vi "mainPLC.vi"(8 "Error In":errorcluster, 11 "plcUDE":T1) -> (0 "Error Out":errorcluster)   [LabVIEW 2018]
uses:
  controls/plcUDE.ctl
  controls/plcData.ctl
  controls/modbusDriverSelectorEnum.ctl
  controls/openModbusConnectionCluster.ctl
  controls/readRegisterModbusCluster.ctl
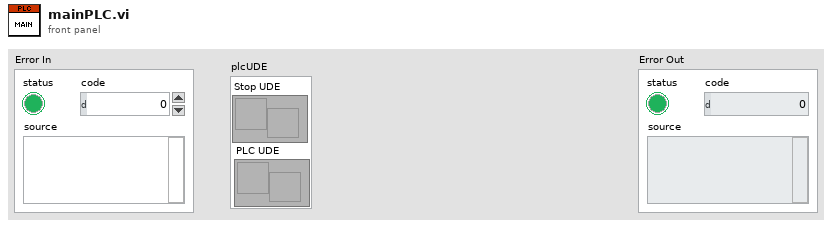
[diagram p1: front panel]
types:
  T1 = typedef "plcUDE.ctl" = cluster{"Stop UDE":refnum<user-event>, "PLC UDE":refnum<user-event>}
  T2 = enum32{"Invalid", "Standard", "Closed", "Hidden", "Minimized", "Maximized"}
  T3 = enum32{"invalid app kind", "Development System", "Run Time System", "Student Edition", "Embedded LabVIEW", "Evaluation", "Custom"}
  T4 = typedef "openModbusConnectionCluster.ctl" = cluster{"IP Address":string, "Timeout (ms)":i32, "Port (502)":u16}
  T5 = typedef "modbusDriverSelectorEnum.ctl" = enum16{"open", "write single holding registers", "read holding registers", "close"}
  T6 = typedef "plcData.ctl" = cluster{"IP Address":string, "Timeout":i32, "Port [502]":u16, "isSimulation?":bool, "Model Number":u16}
  T7 = cluster{"Core":cluster{"Current VI Reference":refnum<vi>, "Close Panel on Exit?":bool}, "plcUDE":T1, "PLC Data":T6, "Address":u16, "Registry":i32, "Setting-Registry":u16, "DB file path":path}
  T8 = cluster{"Current VI Reference":refnum<vi>, "Close Panel on Exit?":bool}
  T9 = typedef "pathCluster.ctl" = cluster{"src Folder Path":path, "Controller Module Path":path, "UI Module Path":path, "Model Select Module Path":path, "Barcode Printer Module Path":path, "Barcode Scanner Module Path":path, "Database Module Path":path, "Report Generation Path":path, "Simulation Path":path, "subVIs Folder Path":path, "info Folder Path":path, "config file Path":path, "cutomerLogo Path":path}
  T10 = typedef "readRegisterModbusCluster.ctl" = cluster{"Starting Address":u16, "Number of Inputs":u16}
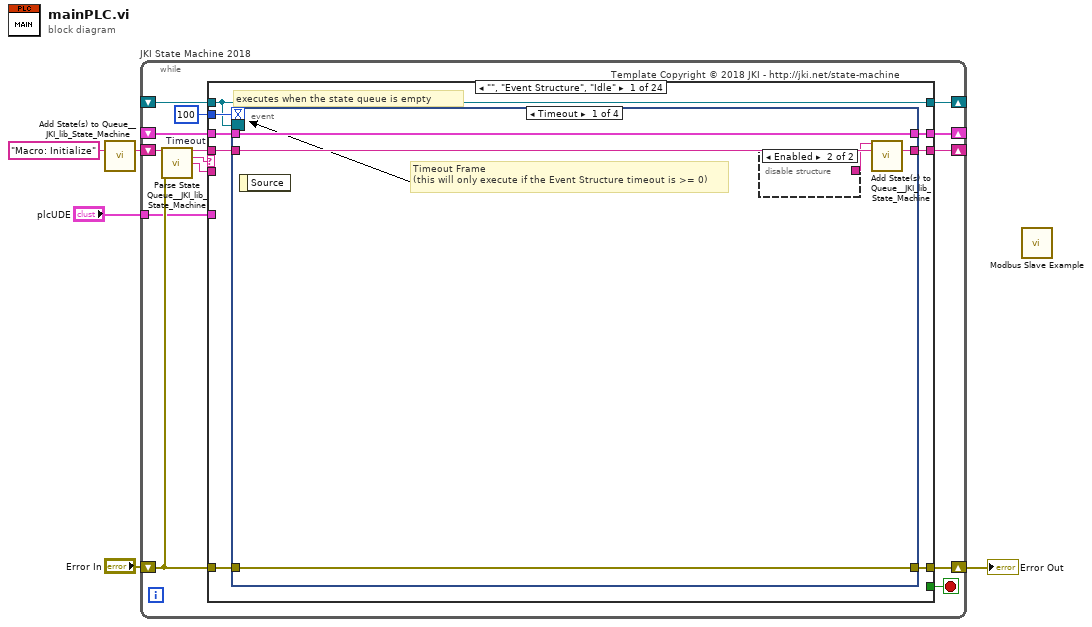
[diagram p0: block diagram]
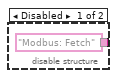
[diagram p2: hidden frame]
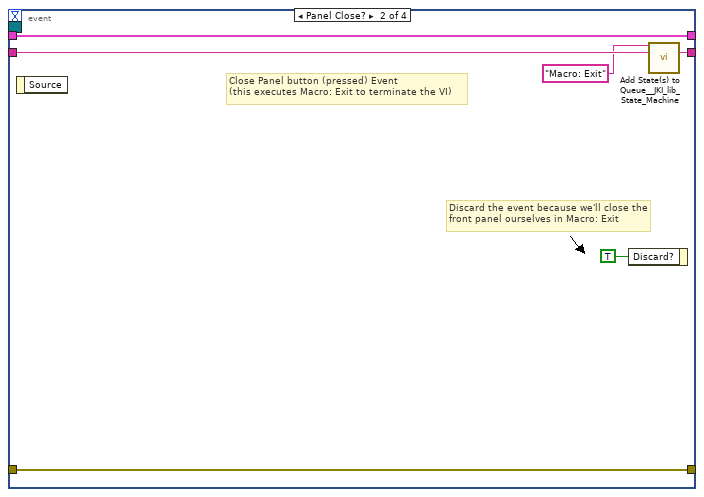
[diagram p3: hidden frame]
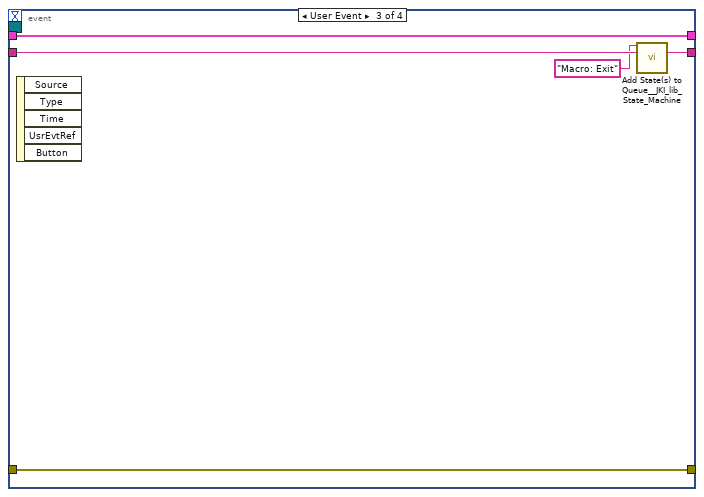
[diagram p4: hidden frame]
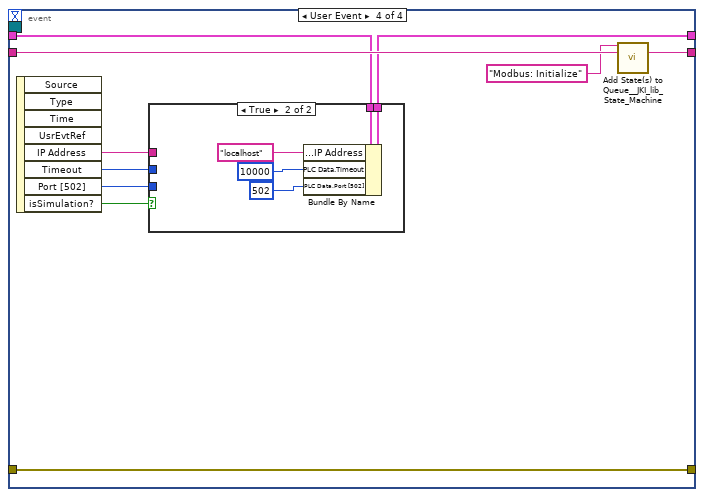
[diagram p5: hidden frame]
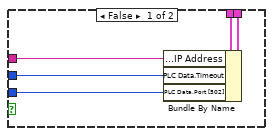
[diagram p6: hidden frame]
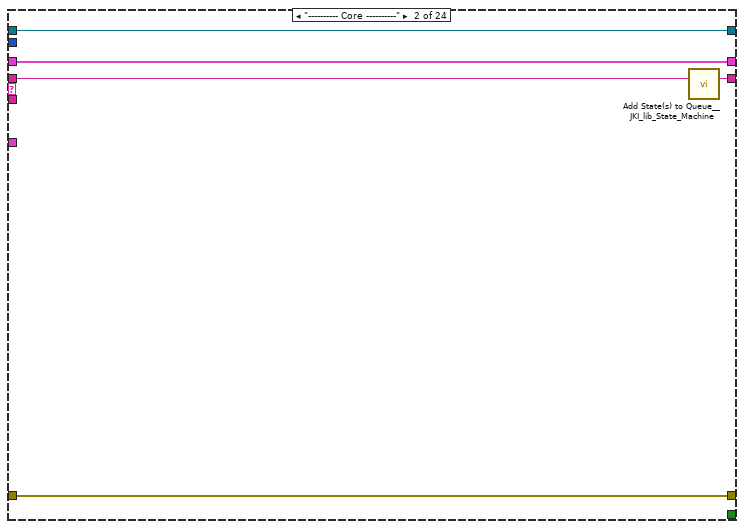
[diagram p7: hidden frame]
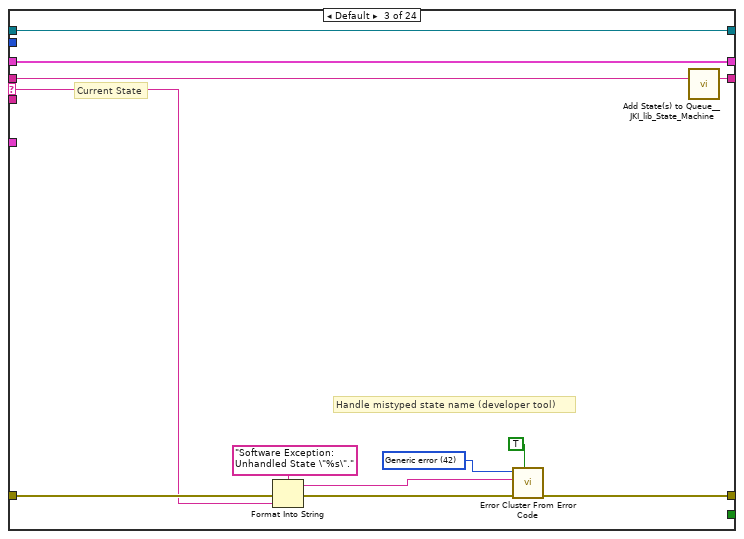
[diagram p8: hidden frame]
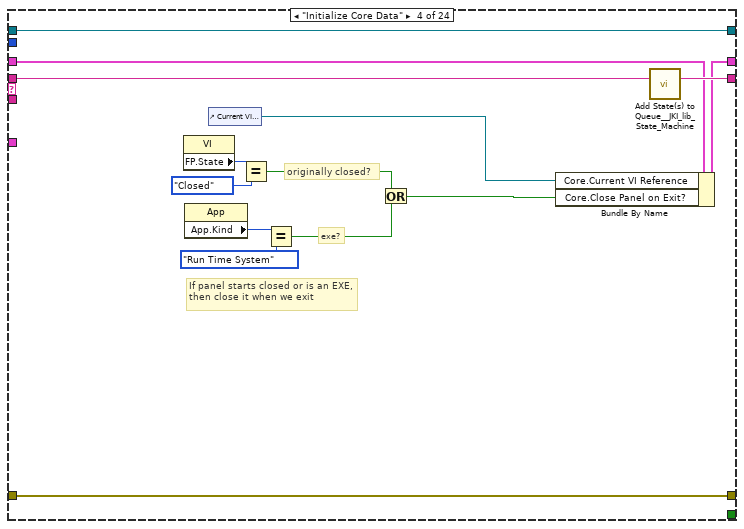
[diagram p9: hidden frame]
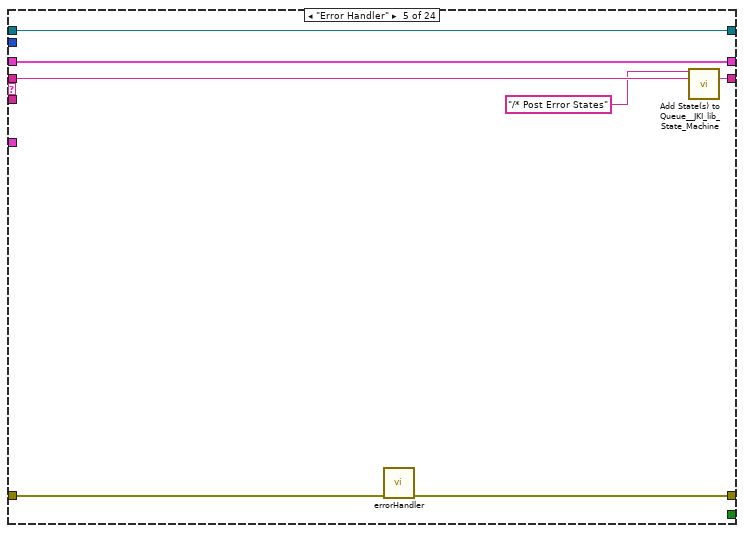
[diagram p10: hidden frame]
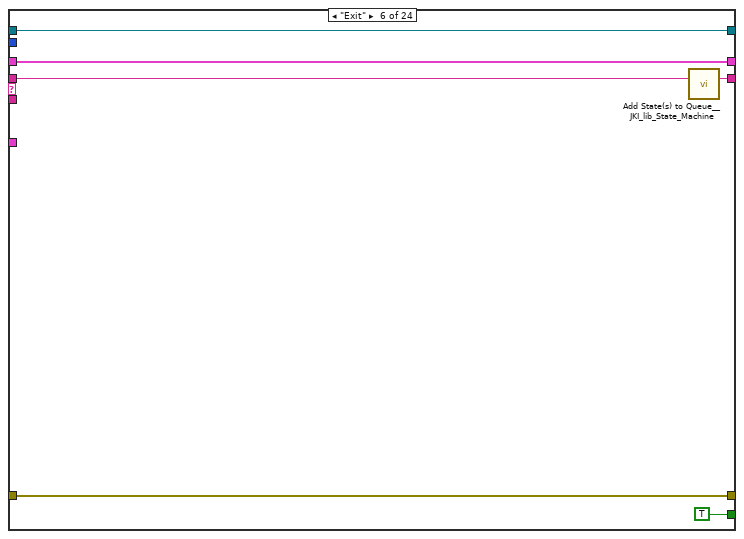
[diagram p11: hidden frame]
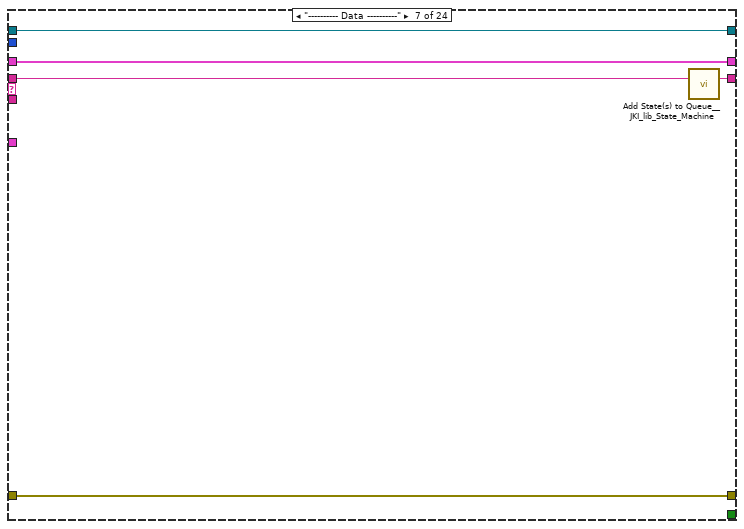
[diagram p12: hidden frame]
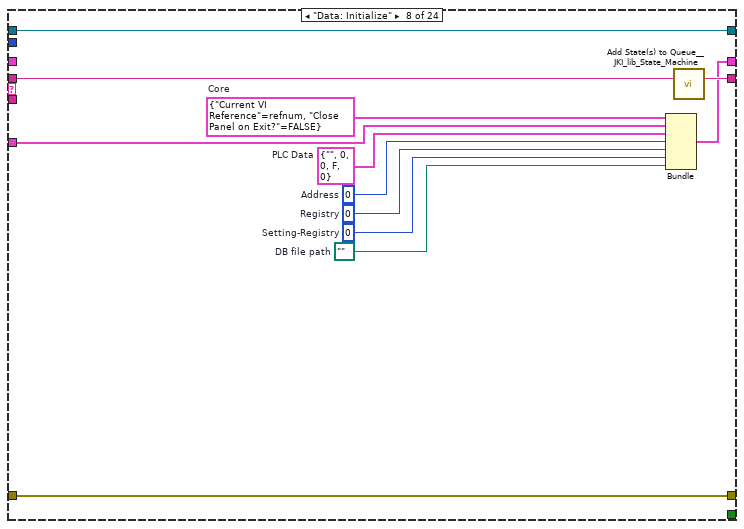
[diagram p13: hidden frame]
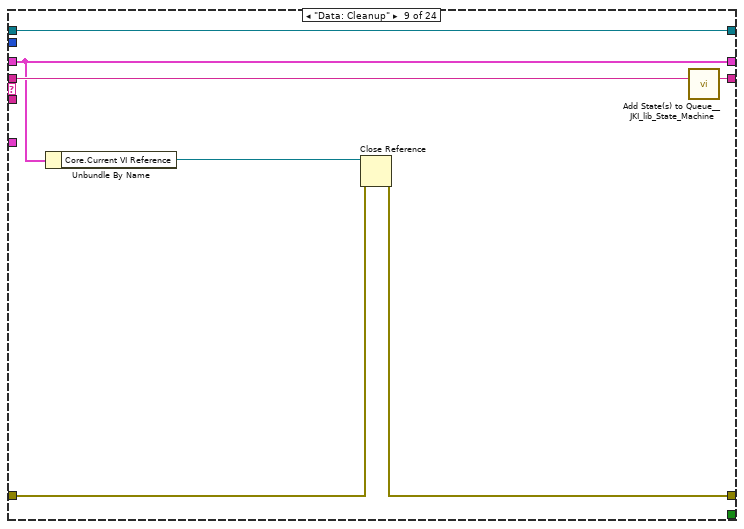
[diagram p14: hidden frame]
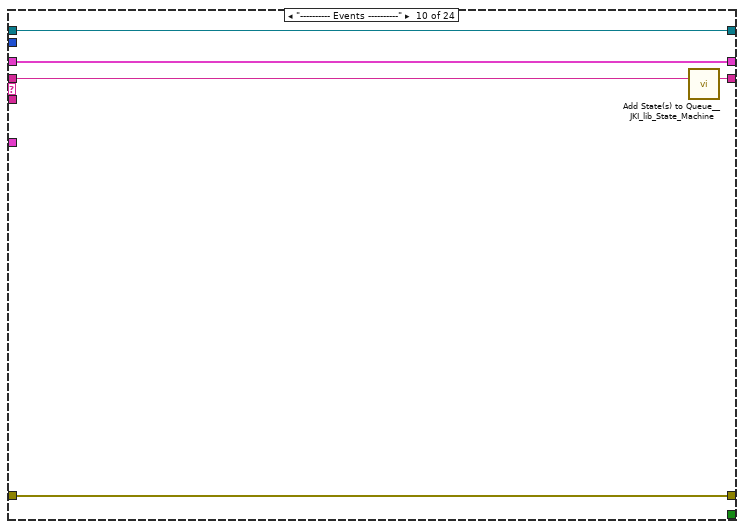
[diagram p15: hidden frame]
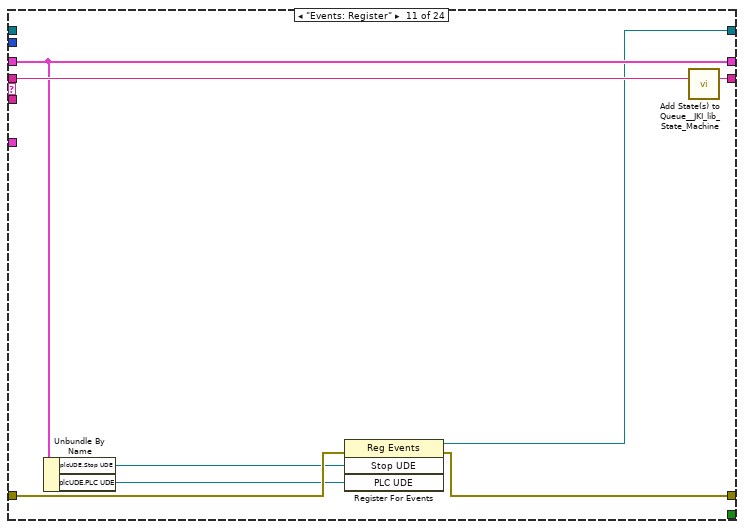
[diagram p16: hidden frame]
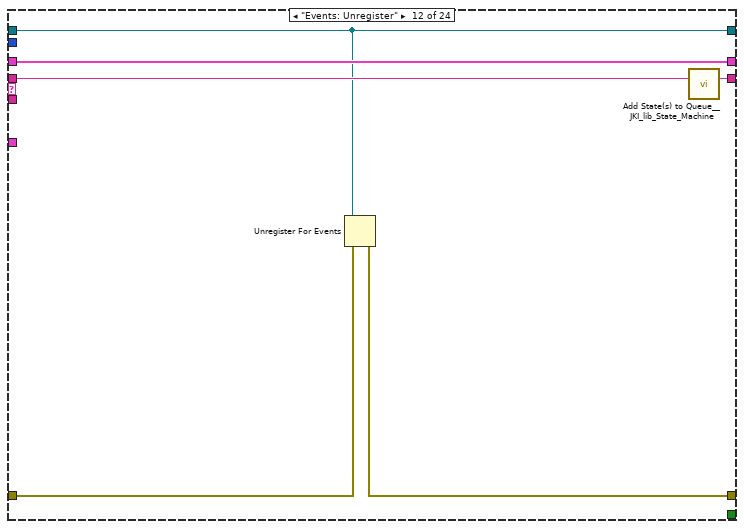
[diagram p17: hidden frame]
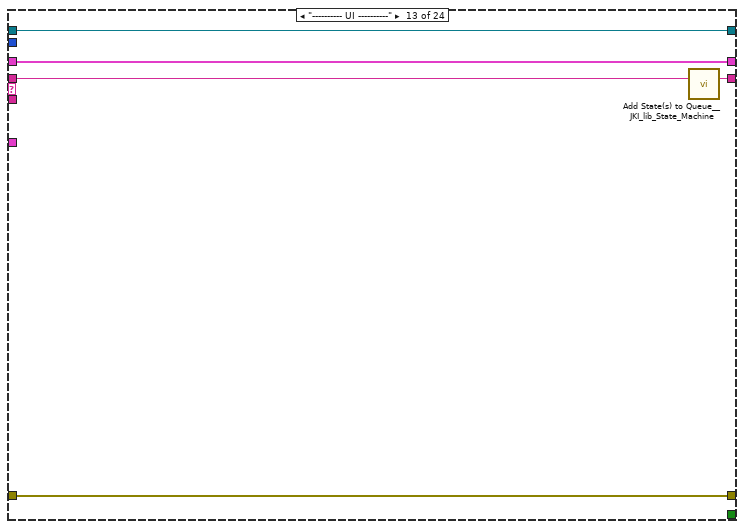
[diagram p18: hidden frame]
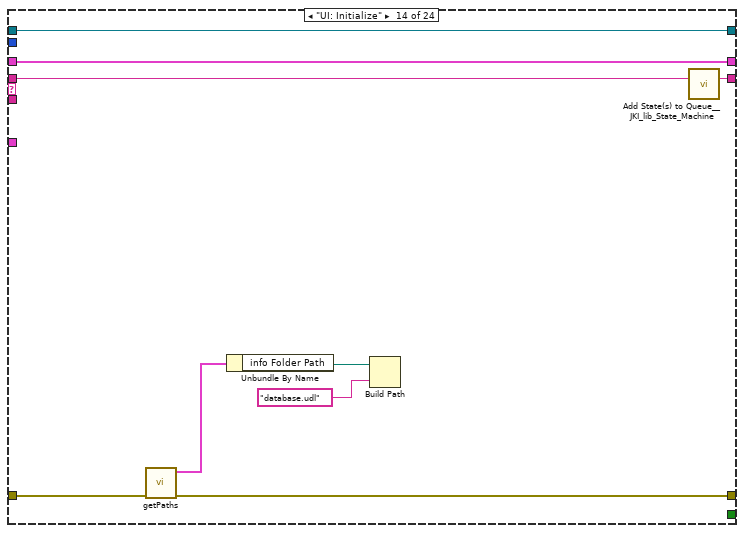
[diagram p19: hidden frame]
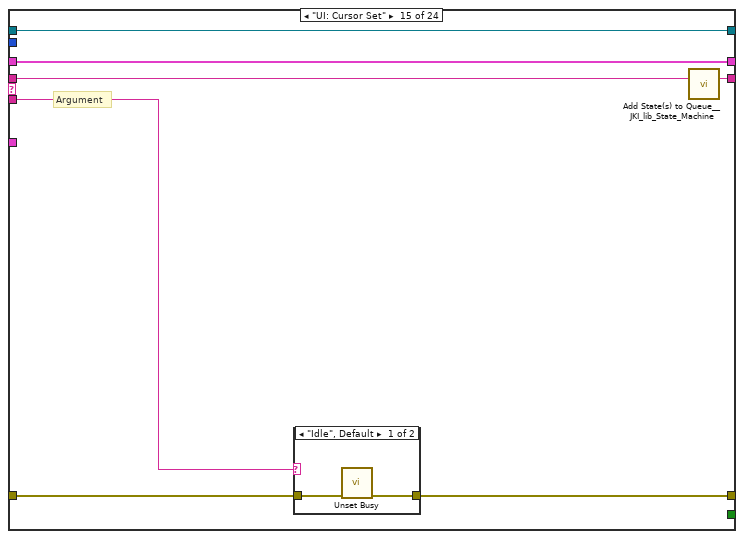
[diagram p20: hidden frame]
diagram:
  n1 = call <vilib>:"Add State(s) to Queue__JKI_lib_State_Machine.vi"("State(s) in (\"\")"="Macro: Initialize") -> ("States Out"=w5:string)  [unwired: 14 in]
  n2 = while "JKI State Machine 2018" {
    shift-right: [w12] -> _
    shift-left: _ -> [w11]
    shift-right: [w15] -> w2
    shift-left: "Error In" -> [w9]
    shift-right: [w14] -> _
    shift-left: w5 -> [w16]
    shift-right: [w8] -> _
    shift-left: _ -> [w7]
    tunnel: "plcUDE" -> [w6]
    stop <- w13 stop-if-true
    w10 = 100  # Timeout
    # "Template Copyright © 2018 JKI - http://jki.net/state-machine"
    n3 = call <vilib>:"Parse State Queue__JKI_lib_State_Machine.vi"("State Queue"=w16, "Error In (no error)"=w9) -> ("Remaining States"=w18:string, "Current State"=w19:string, "Arguments"=w17:string)  [unwired: 11 in]
    n4 = case shown="\"\", \"Event Structure\", \"Idle\"" w19 {
      selector: w19 -> [_ _ w71 _ _ _ _ _ _ _ _ _ _ _ _ _ _ _ _ _ _ _ _ _]
      tunnel: w18 -> [w27 w69 w75 w95 w102 w108 w113 w125 w132 w137 w145 w151 w156 w165 w172 w184 w254 w260 w271 w276 w288 w306 w315 w334]
      tunnel: w17 -> [_ _ _ _ _ _ _ _ _ _ _ _ _ _ w167 w178 _ _ _ _ _ _ _ _]
      tunnel: w11 -> [w25 w66 w73 w88 w100 w106 w110 _ w127 w134 w141 w149 w153 w162 w170 w180 w251 w257 w268 w273 w282 w296 w312 w332]
      tunnel: [w24 w67 w77 w92 w96 w105 w111 w122 w128 w135 w143 w146 w154 w160 w168 w181 w252 w258 w269 w274 w284 w302 w310 w327] -> w15
      tunnel: w9 -> [w23 w67 w76 w92 w97 w105 w111 w122 w129 w135 w142 w147 w154 w161 w169 w182 w252 w258 w269 w274 w285 w303 w311 w330]
      tunnel: [w26 w68 w74 w94 w101 w107 w112 w124 w131 w136 w144 w150 w155 w164 w171 w183 w253 w259 w270 w275 w287 w305 w314 w333] -> w14
      tunnel: [_ _ _ _ _ TRUE _ _ _ _ _ _ _ _ _ _ _ _ _ _ _ _ _ _] -> w13
      tunnel: [w22 w66 w73 w93 w100 w106 w110 w123 w127 w134 w141 w149 w153 w162 w170 w180 w251 w257 w268 w273 w282 w295 w312 w332] -> w12
      tunnel: w10 -> [w21 _ _ _ _ _ _ _ _ _ _ _ _ _ _ _ _ _ _ _ _ _ _ _]
      tunnel: [w20 w65 w70 w82 w98 w103 w109 w120 w126 w133 w138 w148 w152 w163 w166 w177 w250 w255 w261 w272 w286 w304 w313 w331] -> w8
      tunnel: w7 -> [w20 w65 w70 w82 w98 w103 w109 w120 w126 w133 _ w148 w152 w163 w166 w177 w250 w255 w261 w272 w286 w304 w313 w331]
      tunnel: w6 -> [_ _ _ _ _ _ _ w119 _ _ _ _ _ _ _ _ _ _ _ _ _ _ _ _]
      frame "", "Event Structure", "Idle" {
        # "executes when the state queue is empty"
        n5 = event shown="[0] Timeout" {
          selector: w20 -> [_ _ _ _]
          dyn-events: _ -> [_ _ _ _]
          timeout: w21 -> [_ _ _ _]
          tunnel: w27 -> [w32 w39 w42 w53]
          tunnel: [w31 w38 w41 w52] -> w26
          tunnel: w25 -> [w29 w36 w44 w45]
          tunnel: [w30 w37 w43 w54] -> w24
          tunnel: w23 -> [w30 w37 w43 w54]
          tunnel: [w29 w36 w44 w46] -> w22
          event Timeout {
            # "Timeout Frame\n(this will only execute if the Event Structure timeout is >= 0)"
            n6 = event-data() -> ()  [unwired: 1 in, 1 out]
            n7 = disable-structure shown="Enabled" {
              disable-tunnel: ["Modbus: Fetch" ("State(s) in Front (\"\")") _] -> w28
              frame Disabled {
              }
              frame Enabled {
              }
            }
            n8 = call <vilib>:"Add State(s) to Queue__JKI_lib_State_Machine.vi"("State(s) in Front (\"\")"=w28, "State(s) in (\"\")"=w32) -> ("States Out"=w31:string)  [unwired: 13 in]
          }
          event Panel Close? {
            # "Discard the event because we'll close the front panel ourselves in Macro: Exit"
            # "Close Panel button (pressed) Event\n(this executes Macro: Exit to terminate the VI)"
            n9 = event-data() -> ()  [unwired: 1 in, 1 out]
            n10 = event-data("Discard?"=TRUE) -> ()  [unwired: 1 in, 1 out]
            n11 = call <vilib>:"Add State(s) to Queue__JKI_lib_State_Machine.vi"("State(s) in Front (\"\")"="Macro: Exit", "State(s) in (\"\")"=w39) -> ("States Out"=w38:string)  [unwired: 13 in]
          }
          event User Event {
            n12 = event-data() -> ()  [unwired: 1 in, 5 out]
            n13 = call <vilib>:"Add State(s) to Queue__JKI_lib_State_Machine.vi"("State(s) in Front (\"\")"="Macro: Exit" ("State(s) in Front (\"\")"), "State(s) in (\"\")"=w42) -> ("States Out"=w41:string)  [unwired: 13 in]
          }
          event User Event {
            n14 = event-data() -> ("IP Address"=w47:string, "Timeout"=w48:i32, "Port [502]"=w49:u16, "isSimulation?"=w50:bool)  [unwired: 1 in, 4 out]
            n15 = case shown="True" w50 {
              tunnel: w49 -> [w57 _]
              tunnel: w48 -> [w58 _]
              tunnel: w47 -> [w59 _]
              tunnel: w45 -> [w56 w64]
              tunnel: [w55 w63] -> w46
              frame False {
                n16 = Bundle By Name(cluster=w56, "PLC Data.IP Address"=w59, "PLC Data.Timeout"=w58, "PLC Data.Port [502]"=w57) -> (w55:T7)
              }
              frame True {
                n17 = Bundle By Name(cluster=w64, "PLC Data.IP Address"="localhost", "PLC Data.Timeout"=10000, "PLC Data.Port [502]"=u16 502) -> (w63:T7)
              }
            }
            n18 = call <vilib>:"Add State(s) to Queue__JKI_lib_State_Machine.vi"("State(s) in Front (\"\")"="Modbus: Initialize" ("State(s) in (\"\")"), "State(s) in (\"\")"=w53) -> ("States Out"=w52:string)  [unwired: 13 in]
          }
        }
      }
      frame "---------- Core ----------" {
        n19 = call <vilib>:"Add State(s) to Queue__JKI_lib_State_Machine.vi"("State(s) in (\"\")"=w69) -> ("States Out"=w68:string)  [unwired: 14 in]
      }
      frame Default {
        w80 = 42 items=["No error", "Argument error", "Memory is full", "Out of zone", "End of file", "File already open", "Generic file I/O error", "File not found", "File permission error", "Disk is full", "Duplicate path", "Too many files open", "System feature not enabled", "Resource file not found", "Cannot add resource", "Resource not found", "Image not found", "Image memory error", "Pen does not exist", "Config type invalid", "Config token not found", "Config parse error", "Config memory error", "Bad external code format", "Bad external code offset", "External code not present", "Null window", "Destroy window error", "Null menu", "Print aborted", "Bad print record", "Print driver error", "Windows error during printing", "Memory error during printing", "Print dialog error", "Generic print error", "Invalid device refnum", "Device not found", "Device parameter error", "Device unit error", "Cannot open device", "Device call aborted", "Generic error", "Cancelled by user", "Object ID too low", "Object ID too high", "Object not in heap", "Unknown heap", "Unknown object (invalid DefProc)", "Unknown object (DefProc not in table)", "Message out of range", "Invalid (null) method", "Unknown message", "Manager call not supported", "Bad address", "Network operation in progress", "Network operation timed out", "Connection is busy", "Network attribute not supported", "Network error", "Address in use", "System out of memory", "Connection aborted", "Connection refused", "Not connected", "Already connected", "Connection closed", "Initialization error (interapplication manager)", "Bad occurrence", "Wait on unbound occurrence handler", "Occurrence queue overflow", "Datalog type conflict", "Unused", "Unrecognized type (interapplication manager)", "Memory corrupt", "Failed to make temporary DLL", "Old CIN version", "Drag socket not found", "Failed to load drop-object", "Failed to register OLE object", "Failed to release OLE object", "Format specifier type mismatch", "Unknown format specifier", "Too few format specifiers", "Too many format specifiers", "Scan failed", "Newer CIN version", "Error converting to variant", "Runtime menu error", "Password tampered", "Variant attribute not found", "Incompatible variant data type", "Event data is not available", "Event Store is not present", "Occurrence is not found", "Event Queue is not created", "Event info is not available", "Refnum passed is NULL", "Error retrieving Class GUID", "Error retrieving CoClass GUID", "Error retrieving TypeLib GUID.", "Bad built application magic bytes.", "Specific driver is different from the specific driver associated with the Logical Name.", "There is no session opened to the class driver.", "Max Error", "MAX - Error with config objects", "MAX - Error loading configuration", "MAX - Group not supported"]
        # "Current State"
        # "Handle mistyped state name (developer tool)"
        n20 = Format Into String(format string="Software Exception: Unhandled State \"%s\"." ("message"), error in=w76, w71) -> (resulting string=w79:string, error out=w78:errorcluster)  [unwired: 1 in]
        n21 = call <vilib>:"Error Cluster From Error Code.vi"("show call chain? (False)"=TRUE, "error in (no error)"=w78, "error message (\"\")"=w79, "error code (0)"=w80) -> ("error out"=w77:errorcluster)  [unwired: 5 in]
        n22 = call <vilib>:"Add State(s) to Queue__JKI_lib_State_Machine.vi"("State(s) in (\"\")"=w75) -> ("States Out"=w74:string)  [unwired: 14 in]
      }
      frame "Initialize Core Data" {
        # "originally closed?"
        # "exe?"
        # "If panel starts closed or is an EXE, then close it when we exit"
        n23 = property class="VI"() -> ("FP.State"=w85:T2)  [unwired: 2 in, 2 out]
        n24 = property class="App"() -> ("App.Kind"=w91:T3)  [unwired: 2 in, 2 out]
        n25 = control-ref of="Current VI Reference"() -> (w86:refnum<vi>)
        n26 = Equal?(x=w85, y=T2."Closed" ("Front Panel Window:State")) -> (x = y?=w83:bool)
        n27 = Equal?(x=w91, y=T3."Run Time System" ("Application:Kind")) -> (x = y?=w89:bool)
        n28 = Or(x=w83, y=w89) -> (x .or. y?=w87:bool)
        n29 = Bundle By Name(cluster=w88, "Core.Current VI Reference"=w86, "Core.Close Panel on Exit?"=w87) -> (w93:T7)
        n30 = call <vilib>:"Add State(s) to Queue__JKI_lib_State_Machine.vi"("State(s) in (\"\")"=w95) -> ("States Out"=w94:string)  [unwired: 14 in]
      }
      frame "Error Handler" {
        n31 = call "errorHandler.vi"("Error In"=w97) -> ("Error Out"=w96:errorcluster)  [unwired: 10 in]
        n32 = call <vilib>:"Add State(s) to Queue__JKI_lib_State_Machine.vi"("State(s) in Front (\"\")"="/* Post Error States", "State(s) in (\"\")"=w102) -> ("States Out"=w101:string)  [unwired: 13 in]
      }
      frame "Exit" {
        n33 = call <vilib>:"Add State(s) to Queue__JKI_lib_State_Machine.vi"("State(s) in (\"\")"=w108) -> ("States Out"=w107:string)  [unwired: 14 in]
      }
      frame "---------- Data ----------" {
        n34 = call <vilib>:"Add State(s) to Queue__JKI_lib_State_Machine.vi"("State(s) in (\"\")"=w113) -> ("States Out"=w112:string)  [unwired: 14 in]
      }
      frame "Data: Initialize" {
        w114 = path ""  # DB file path
        w115 = u16 0  # Setting-Registry
        w116 = 0  # Registry
        w117 = u16 0  # Address
        w118 = T6 {"IP Address"="", "Timeout"=0, "Port [502]"=0, "isSimulation?"=FALSE, "Model Number"=0}  # PLC Data
        w121 = T8 {"Current VI Reference"=refnum, "Close Panel on Exit?"=FALSE}  # Core
        n35 = Bundle("Core"=w121, "plcUDE"=w119, "PLC Data"=w118, "Address"=w117, "Registry"=w116, "Setting-Registry"=w115, "DB file path"=w114) -> (w123:T7)  [unwired: 1 in]
        n36 = call <vilib>:"Add State(s) to Queue__JKI_lib_State_Machine.vi"("State(s) in (\"\")"=w125) -> ("States Out"=w124:string)  [unwired: 14 in]
      }
      frame "Data: Cleanup" {
        n37 = Unbundle By Name(w127) -> ("Core.Current VI Reference"=w130:refnum<vi>)
        n38 = Close Reference(reference=w130, error in (no error)=w129) -> (error out=w128:errorcluster)
        n39 = call <vilib>:"Add State(s) to Queue__JKI_lib_State_Machine.vi"("State(s) in (\"\")"=w132) -> ("States Out"=w131:string)  [unwired: 14 in]
      }
      frame "---------- Events ----------" {
        n40 = call <vilib>:"Add State(s) to Queue__JKI_lib_State_Machine.vi"("State(s) in (\"\")"=w137) -> ("States Out"=w136:string)  [unwired: 14 in]
      }
      frame "Events: Register" {
        n41 = Unbundle By Name(w141) -> ("plcUDE.Stop UDE"=w140:refnum<user-event>, "plcUDE.PLC UDE"=w139:refnum<user-event>)
        n42 = register-events(error in=w142, w140, w139) -> (reference out=w138:refnum<event-registration>, error out=w143:errorcluster)  [unwired: 1 in]
        n43 = call <vilib>:"Add State(s) to Queue__JKI_lib_State_Machine.vi"("State(s) in (\"\")"=w145) -> ("States Out"=w144:string)  [unwired: 14 in]
      }
      frame "Events: Unregister" {
        n44 = Unregister For Events(event registration refnum=w148, error in=w147) -> (error out=w146:errorcluster)
        n45 = call <vilib>:"Add State(s) to Queue__JKI_lib_State_Machine.vi"("State(s) in (\"\")"=w151) -> ("States Out"=w150:string)  [unwired: 14 in]
      }
      frame "---------- UI ----------" {
        n46 = call <vilib>:"Add State(s) to Queue__JKI_lib_State_Machine.vi"("State(s) in (\"\")"=w156) -> ("States Out"=w155:string)  [unwired: 14 in]
      }
      frame "UI: Initialize" {
        n47 = call "getPaths.vi"("Error In"=w161) -> ("Error Out"=w160:errorcluster, "Application Path Cluster"=w159:T9)  [unwired: 9 in]
        n48 = Unbundle By Name(w159) -> ("info Folder Path"=w158:path)
        n49 = Build Path(base path=w158, name or relative path="database.udl") -> ()  [unwired: 1 out]
        n50 = call <vilib>:"Add State(s) to Queue__JKI_lib_State_Machine.vi"("State(s) in (\"\")"=w165) -> ("States Out"=w164:string)  [unwired: 14 in]
      }
      frame "UI: Cursor Set" {
        # "Argument"
        n51 = case shown="\"Idle\", Default" w167 {
          tunnel: w169 -> [w174 w176]
          tunnel: [w173 w175] -> w168
          frame "Idle", Default {
            n52 = call <vilib>:"Unset Busy.vi"("error in (no error)"=w174) -> ("error out"=w173:errorcluster)  [unwired: 10 in]
          }
          frame "Busy" {
            n53 = call <vilib>:"Set Busy.vi"("error in (no error)"=w176) -> ("error out"=w175:errorcluster)  [unwired: 9 in, 1 out]
          }
        }
        n54 = call <vilib>:"Add State(s) to Queue__JKI_lib_State_Machine.vi"("State(s) in (\"\")"=w172) -> ("States Out"=w171:string)  [unwired: 14 in]
      }
      frame "UI: Front Panel State" {
        # "Argument"
        n55 = Unbundle By Name(w180) -> ("Core.Current VI Reference"=w179:refnum<vi>)
        n56 = case shown="\"Open\", \"Standard\", Default" w178 {
          tunnel: w182 -> [w190 w205 w216 w229 w242]
          tunnel: [w192 w206 w218 w231 w244] -> w181
          tunnel: w179 -> [w191 w203 w217 w230 w243]
          frame "Open", "Standard", Default {
            w185 = T2."Hidden" ("State")
            n57 = property class="VI"(reference=w191, error in=w190) -> (reference out=w188:refnum<vi>, error out=w189:errorcluster, "FP.State"=w187:T2)
            n58 = Not Equal?(x=w187, y=w185) -> (x != y?=w186:bool)
            n59 = case shown="True" w186 {
              tunnel: [w196 w198] -> w192
              tunnel: w189 -> [w195 w198]
              tunnel: w188 -> [w194 _]
              tunnel: w185 -> [w193 _]
              frame True {
                n60 = invoke class="VI" method="FP.Open"(reference=w194, error in=w195, "Activate"=TRUE, "State"=w193) -> (error out=w196:errorcluster)  [unwired: 1 in, 4 out]
              }
              frame False {
              }
            }
          }
          frame "Close", "Closed" {
            n61 = property class="VI"(reference=w203, error in=w205) -> (reference out=w202:refnum<vi>, error out=w204:errorcluster, "FP.State"=w200:T2)
            n62 = Not Equal?(x=w200, y=T2."Closed" ("Front Panel Window:State")) -> (x != y?=w199:bool)
            n63 = case shown="True" w199 {
              tunnel: [w207 w210] -> w206
              tunnel: w204 -> [w207 w209]
              tunnel: w202 -> [_ w208]
              frame False {
              }
              frame True {
                n64 = invoke class="VI" method="FP.Close"(reference=w208, error in=w209) -> (error out=w210:errorcluster)  [unwired: 1 in, 2 out]
              }
            }
          }
          frame "Hidden", "Hide" {
            w211 = T2."Hidden" ("State")
            n65 = property class="VI"(reference=w217, error in=w216) -> (reference out=w214:refnum<vi>, error out=w215:errorcluster, "FP.State"=w213:T2)
            n66 = Not Equal?(x=w213, y=w211) -> (x != y?=w212:bool)
            n67 = case shown="True" w212 {
              tunnel: [w222 w223] -> w218
              tunnel: w215 -> [w221 w223]
              tunnel: w214 -> [w220 _]
              tunnel: w211 -> [w219 _]
              frame True {
                n68 = invoke class="VI" method="FP.Open"(reference=w220, error in=w221, "State"=w219) -> (error out=w222:errorcluster)  [unwired: 2 in, 4 out]
              }
              frame False {
              }
            }
          }
          frame "Minimize", "Minimized" {
            w224 = T2."Minimized" ("State")
            n69 = property class="VI"(reference=w230, error in=w229) -> (reference out=w227:refnum<vi>, error out=w228:errorcluster, "FP.State"=w226:T2)
            n70 = Not Equal?(x=w226, y=w224) -> (x != y?=w225:bool)
            n71 = case shown="True" w225 {
              tunnel: [w235 w236] -> w231
              tunnel: w228 -> [w234 w236]
              tunnel: w227 -> [w233 _]
              tunnel: w224 -> [w232 _]
              frame True {
                n72 = invoke class="VI" method="FP.Open"(reference=w233, error in=w234, "State"=w232) -> (error out=w235:errorcluster)  [unwired: 2 in, 4 out]
              }
              frame False {
              }
            }
          }
          frame "Maximize", "Maximized" {
            w237 = T2."Maximized" ("State")
            n73 = property class="VI"(reference=w243, error in=w242) -> (reference out=w240:refnum<vi>, error out=w241:errorcluster, "FP.State"=w239:T2)
            n74 = Not Equal?(x=w239, y=w237) -> (x != y?=w238:bool)
            n75 = case shown="True" w238 {
              tunnel: [w248 w249] -> w244
              tunnel: w241 -> [w247 w249]
              tunnel: w240 -> [w246 _]
              tunnel: w237 -> [w245 _]
              frame True {
                n76 = invoke class="VI" method="FP.Open"(reference=w246, error in=w247, "State"=w245) -> (error out=w248:errorcluster)  [unwired: 2 in, 4 out]
              }
              frame False {
              }
            }
          }
        }
        n77 = call <vilib>:"Add State(s) to Queue__JKI_lib_State_Machine.vi"("State(s) in (\"\")"=w184) -> ("States Out"=w183:string)  [unwired: 14 in]
      }
      frame "---------- Macro ----------" {
        n78 = call <vilib>:"Add State(s) to Queue__JKI_lib_State_Machine.vi"("State(s) in (\"\")"=w254) -> ("States Out"=w253:string)  [unwired: 14 in]
      }
      frame "Macro: Initialize" {
        n79 = call <vilib>:"Add State(s) to Queue__JKI_lib_State_Machine.vi"("State(s) in Front (\"\")"="Data: Initialize\nInitialize Core Data\nEvents: Register\nUI: Initialize\nUI: Front Panel State >> Open", "State(s) in (\"\")"=w260) -> ("States Out"=w259:string)  [unwired: 13 in]
      }
      frame "Macro: Exit" {
        n80 = Unbundle By Name(w268) -> ("Core.Close Panel on Exit?"=w267:bool)
        n81 = Select(t="UI: Front Panel State >> Close", s=w267, f="") -> (s? t:f=w264:string)
        n82 = call <vilib>:"Add State(s) to Queue__JKI_lib_State_Machine.vi"("State(s) in (\"\")"=w264, "State(s) at Back (\"\")"="Modbus: Close\nData: Cleanup\nEvents: Unregister\nExit") -> ("States Out"=w262:string)  [unwired: 13 in]
        n83 = call <vilib>:"Add State(s) to Queue__JKI_lib_State_Machine.vi"("State(s) in Front (\"\")"=w262, "State(s) in (\"\")"=w271) -> ("States Out"=w270:string)  [unwired: 13 in]
      }
      frame "---------- Modbus ----------" {
        n84 = call <vilib>:"Add State(s) to Queue__JKI_lib_State_Machine.vi"("State(s) in (\"\")"=w276) -> ("States Out"=w275:string)  [unwired: 14 in]
      }
      frame "Modbus: Initialize" {
        n85 = Unbundle By Name(w282) -> ("PLC Data.IP Address"=w279:string, "PLC Data.Timeout"=w277:i32, "PLC Data.Port [502]"=w278:u16)
        n86 = Bundle By Name(cluster=T4 {"IP Address"="", "Timeout (ms)"=0, "Port (502)"=0} ("Open Modbus Connection Cluster"), "IP Address"=w279, "Timeout (ms)"=w277, "Port (502)"=w278) -> (w280:T4)
        n87 = call "modbusTCPMasterDriver.vi"("Modbus Driver Selector Enum"=modbusDriverSelectorEnum."open", "Error In"=w285, "Open Modbus Connection Cluster"=w280) -> ("Error Out"=w284:errorcluster)  [unwired: 7 in, 1 out]
        n88 = call <vilib>:"Add State(s) to Queue__JKI_lib_State_Machine.vi"("State(s) in (\"\")"=w288) -> ("States Out"=w287:string)  [unwired: 14 in]
      }
      frame "Modbus: Fetch" {
        w291 = T10 {"Starting Address"=0, "Number of Inputs"=1} ("Read Modbus Register")
        n89 = Unbundle By Name(w296) -> ("Setting-Registry"=w299:u16)
        n90 = call "modbusTCPMasterDriver.vi"("Modbus Driver Selector Enum"=modbusDriverSelectorEnum."read holding registers", "Error In"=w303, "Read Modbus Register"=w291) -> ("Error Out"=w302:errorcluster, "Register Value"=w301:u16[])  [unwired: 7 in]
        n91 = Unbundle By Name(w291) -> ("Starting Address"=w290:u16)
        n92 = Index Array(array=w301, index=0) -> (element=w294:u16)
        n93 = Not Equal?(x=w299, y=w294) -> (x != y?=w298:bool)
        n94 = Select(t="Modbus: Decide", s=w298, f="") -> (s? t:f=w293:string)
        n95 = Bundle By Name(cluster=w296, "Address"=w290, "Setting-Registry"=w294) -> (w295:T7)
        n96 = call <vilib>:"Add State(s) to Queue__JKI_lib_State_Machine.vi"("State(s) in Front (\"\")"=w293, "State(s) in (\"\")"=w306) -> ("States Out"=w305:string)  [unwired: 13 in]
      }
      frame "Modbus: Decide" {
        n97 = Unbundle By Name(w312) -> ("Address"=w309:u16, "Registry"=w308:i32, "DB file path"=w307:path)
        n98 = case shown="0, Default" w309 {
          tunnel: w311 -> [w319 w326]
          tunnel: [w318 w326] -> w310
          tunnel: w308 -> [w317 _]
          tunnel: w307 -> [w316 _]
          frame 0, Default {
            n99 = case shown="1" w317 {
              selector: w317 -> [_ w322]
              tunnel: w319 -> [w321 w325]
              tunnel: [w321 w324] -> w318
              tunnel: w316 -> [_ w323]
              frame 0, Default {
                n100 = One Button Dialog(message="No valid model!") -> ()  [unwired: 1 in, 1 out]
              }
              frame 1 {
                n101 = call "updateModelNumber.vi"("Error In"=w325, "Model Number"=w322, "DB File Path"=w323) -> ("Error Out"=w324:errorcluster)  [unwired: 8 in]
              }
            }
          }
          frame 1 {
          }
        }
        n102 = call <vilib>:"Add State(s) to Queue__JKI_lib_State_Machine.vi"("State(s) in (\"\")"=w315) -> ("States Out"=w314:string)  [unwired: 14 in]
      }
      frame "Modbus: Close" {
        n103 = call "modbusTCPMasterDriver.vi"("Modbus Driver Selector Enum"=modbusDriverSelectorEnum."close", "Error In"=w330) -> ("Error Out"=w328:errorcluster)  [unwired: 8 in, 1 out]
        n104 = call <vilib>:"Clear Errors.vi"("error in (no error)"=w328) -> ("error out"=w327:errorcluster)  [unwired: 5 in, 1 out]
        n105 = call <vilib>:"Add State(s) to Queue__JKI_lib_State_Machine.vi"("State(s) in (\"\")"=w334) -> ("States Out"=w333:string)  [unwired: 14 in]
      }
    }
  }
  "Error Out" <- w2
  n106 = call <vilib>:"Modbus Slave Example.vi"() -> ()  [unwired: 12 in]
